vi "OFF_Polarity_Channel.vi"(5 "CH_ON:0/OFF:1":u16, 7 "Mode":u16(ring)=1 items=["Tx"=1, "Rx"=2], 8 "error in":errorcluster, 11 "TCPIPin":T1={"address"="192.168.100.111", "remote port or service name"=5025, "timeout ms (60000)"=10000}) -> (0 "error out":errorcluster, 1 "OK?":bool, 3 "TCPIPout":T1={"address"="192.168.100.111", "remote port or service name"=5025, "timeout ms (60000)"=10000})   [LabVIEW 2023]
panel:
  out "Array":string[][](array[string])
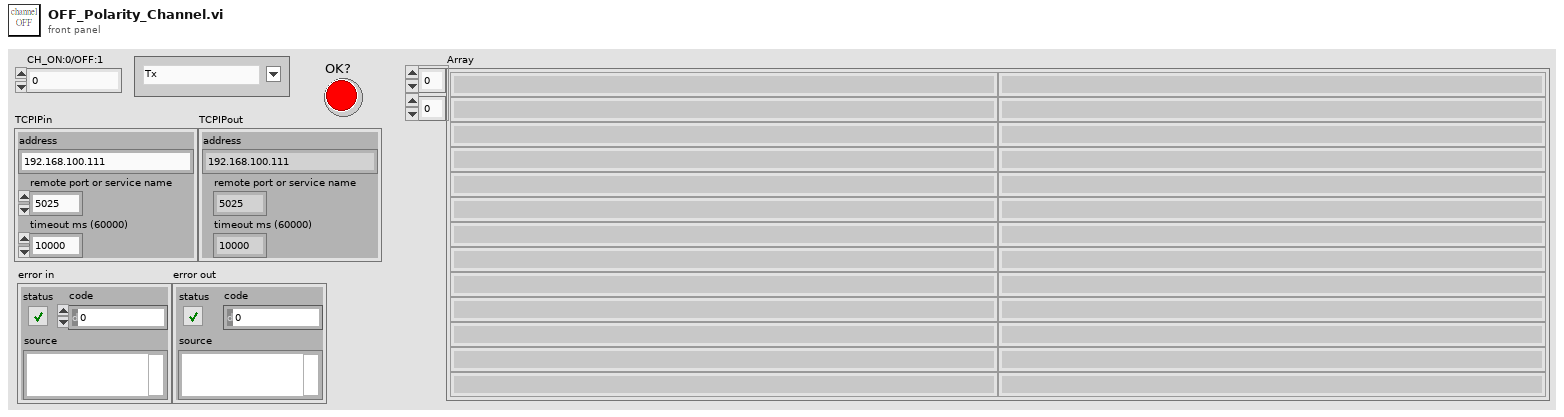
[diagram p1: front panel]
types:
  T1 = cluster{"address":string, "remote port or service name":u16, "timeout ms (60000)":i32}
  T2 = cluster{"Mode":u16, "Polarity":u16, "CH_ON/OFF":u16, "Channel":i32, "Gain":i32, "Phase":i32}
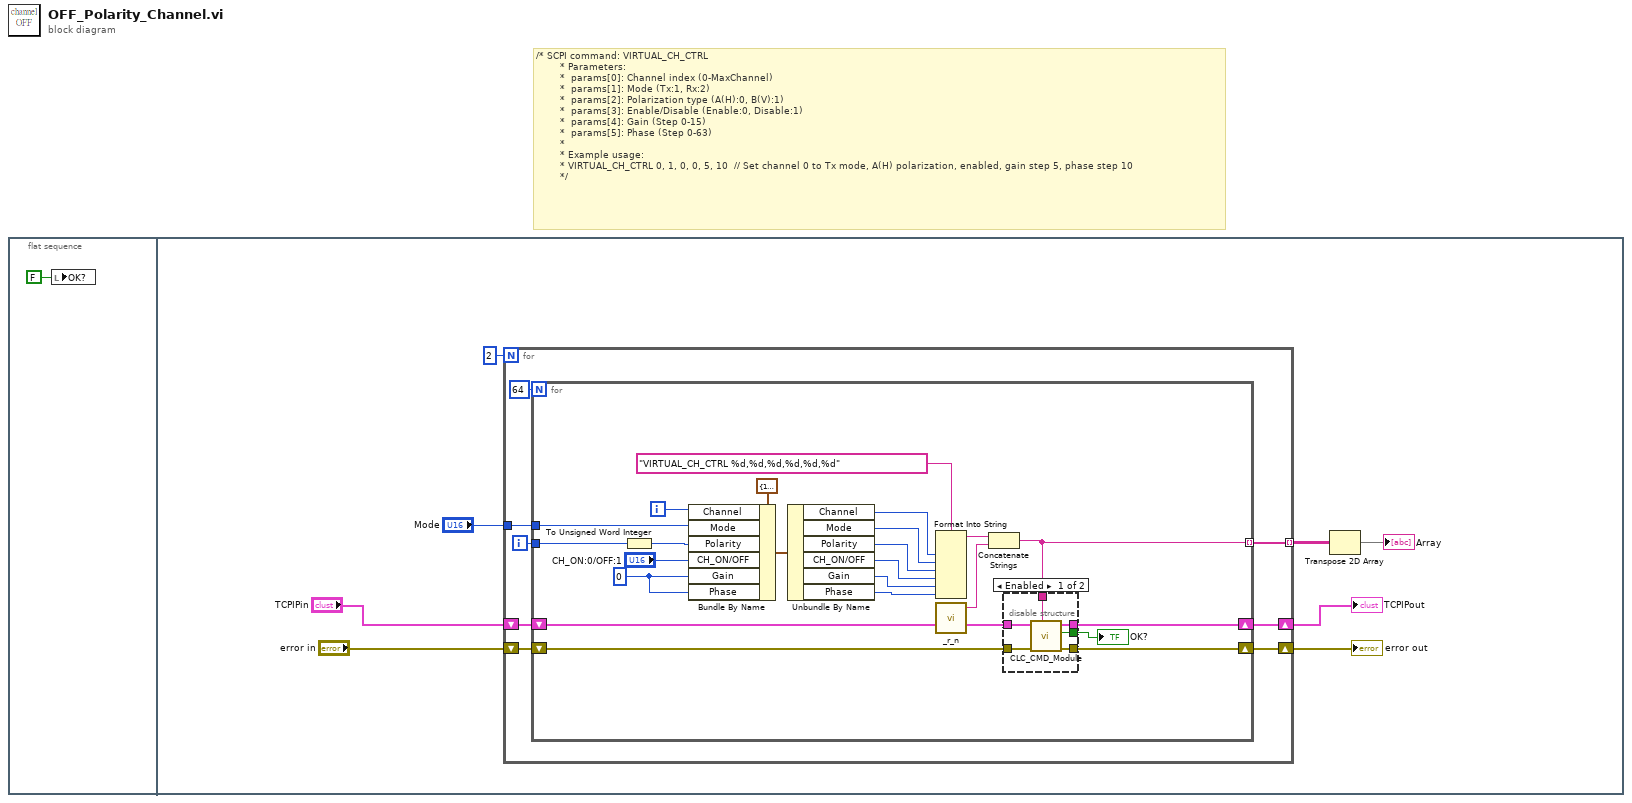
[diagram p0: block diagram]
diagram:
  # "/* SCPI command: VIRTUAL_CH_CTRL\n        * Parameters:\n        *  params[0]: Channel index (0-MaxChannel)\n        *  params[1]: Mode (Tx:1, Rx:2)\n        *  params[2]: Polarization type (A(H):0, B(V):1)\n        *  params[3]: Enable/Disable (Enable:0, Disable:1)\n        *  params[4]: Gain (Step 0-15)\n        *  params[5]: Phase (Step 0-63)\n        * \n        * Example usage:\n        * VIRTUAL_CH_CTRL 0, 1, 0, 0, 5, 10  // Set channel 0 to Tx mode, A(H) polarization, enabled, gain step 5, phase step 10\n        */"
  n1 = flat-sequence {
    frame #0 {
      n2 = local write "OK?"(FALSE ("OK?")) -> ()
    }
    frame #1 {
      n3 = for {
        N: 2 -> [_]
        shift-right: [w16] -> w8
        shift-left: "TCPIPin" -> [w17]
        shift-right: [w14] -> w6
        shift-left: "error in" -> [w15]
        tunnel: "Mode" -> [w12]
        tunnel: [w10] -> w3 mode=indexing
        i -> [w11]
        n4 = for {
          N: 64 -> [_]
          shift-right: [w39] -> w16
          shift-left: w17 -> [w40]
          shift-right: [w37] -> w14
          shift-left: w15 -> [w38]
          tunnel: w12 -> [w25]
          tunnel: w11 -> [w22]
          tunnel: [w19] -> w10 mode=indexing
          i -> [w23]
          w20 = 0 ("Gain")
          n5 = To Unsigned Word Integer(number=w22) -> (unsigned 16bit integer=w21:u16)
          n6 = Bundle By Name(cluster=T2 {"Mode"=1, "Polarity"=1, "CH_ON/OFF"=1, "Channel"=0, "Gain"=0, "Phase"=0} ("Channel params"), "Channel"=w23, "Mode"=w25, "Polarity"=w21, "CH_ON/OFF"="CH_ON:0/OFF:1", "Gain"=w20, "Phase"=w20) -> (w26:T2)
          n7 = Unbundle By Name(w26) -> ("Channel"=w31:i32, "Mode"=w32:u16, "Polarity"=w33:u16, "CH_ON/OFF"=w34:u16, "Gain"=w35:i32, "Phase"=w36:i32)
          n8 = Format Into String(format string="VIRTUAL_CH_CTRL %d,%d,%d,%d,%d,%d" ("data in"), w31, w32, w33, w34, w35, w36) -> (resulting string=w29:string)  [unwired: 2 in, 1 out]
          n9 = call "_r_n.vi"() -> ("command"=w30:string)  [unwired: 5 in]
          n10 = Concatenate Strings(w29, w30) -> (w19:string)
          n11 = disable-structure shown="Enabled" {
            disable-tunnel: w40 -> [w46 w48]
            disable-tunnel: [w45 w48] -> w39
            disable-tunnel: w38 -> [w44 w47]
            disable-tunnel: [w43 w47] -> w37
            disable-tunnel: w19 -> [w42 _]
            disable-tunnel: [w41 _] -> w24
            frame Enabled {
              n12 = call "CLC_CMD_Module.vi"("CMD in"=w42, "error in"=w44, "TCPIPin"=w46) -> ("error out"=w43:errorcluster, "OK?"=w41:bool, "TCPIPout"=w45:T1)  [unwired: 5 in, 1 out]
            }
            frame Disabled {
            }
          }
          "OK?" <- w24
        }
      }
      "TCPIPout" <- w8
      "error out" <- w6
      n13 = Transpose 2D Array(2D array=w3) -> (transposed array=→"Array":string[][])
    }
  }
